vi "XML - Get General Settings.vi"(8 "error in (no error)":errorcluster, 11 "Target Ref in":T2 format="%.0x") -> (0 "error out":errorcluster, 2 "XML Header Data":T1, 3 "Target Ref out":T2 format="%.0x")   [LabVIEW 2019]
doc: "This VI gets all General Settings information required for the export to the XML File. It includes:\n- Custom-Device Type (Synchronous (UDP) - Asynchronous (TCP))\n- Controller Name\n- System Definition File Version\n- Creation Date."
uses:
  <vilib>/NI VeriStand/Custom Device API/Custom Device Item Ref.ctl
  Types/XML/XML - Header Data.ctl
  <vilib>/NI VeriStand/Custom Device API/Custom Device Pointer.ctl
  NationalInstruments.VeriStand.SystemStorage
  <vilib>/NI VeriStand/Custom Device API/Custom Device API.lvlib
  UDP-Custom-Device System Explorer.lvlib
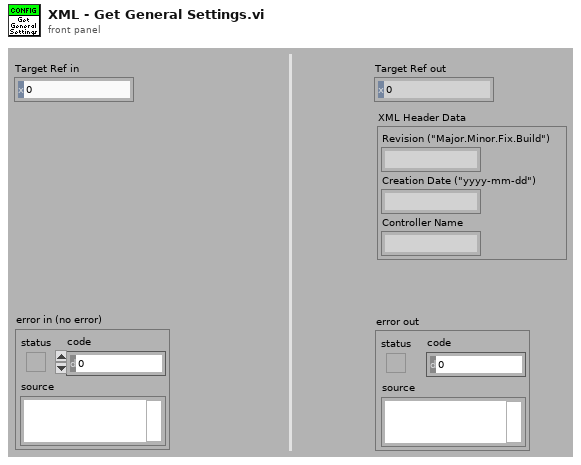
[diagram p1: front panel]
types:
  T1 = typedef "UDP-Custom-Device System Explorer.lvlib/XML - Header Data.ctl" = cluster{"Revision (\"Major.Minor.Fix.Build\")":string, "Creation Date (\"yyyy-mm-dd\")":string, "Controller Name":string}
  T2 = typedef "Custom Device API.lvlib/Custom Device Item Ref.ctl" = u64
  T3 = typedef "Custom Device API.lvlib/Custom Device Pointer.ctl" = refnum<k24>
  T4 = typedef "Custom Device API.lvlib/Custom Device Item Info.ctl" = cluster{"Name":string, "Is Channel":bool, "GUID":string, "Is Waveform":bool}
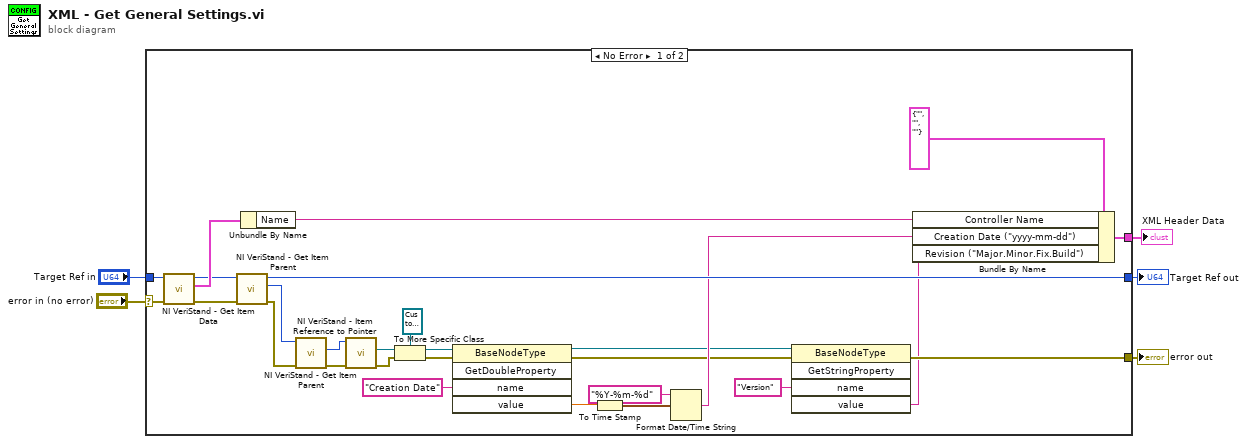
[diagram p0: block diagram]
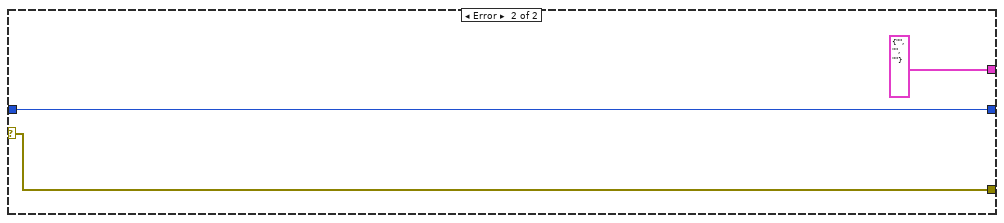
[diagram p2: hidden frame]
diagram:
  n1 = case shown="No Error" "error in (no error)" {
    selector: "error in (no error)" -> [w8 w35]
    tunnel: [w6 T1 {"Revision (\"Major.Minor.Fix.Build\")"="", "Creation Date (\"yyyy-mm-dd\")"="", "Controller Name"=""} ("XML Header Data")] -> w1
    tunnel: "Target Ref in" -> [w22 w36]
    tunnel: [w20 w36] -> w4
    tunnel: [w13 w35] -> w3
    frame No Error {
      n2 = call <vilib>:"NI VeriStand - Get Item Data.vi"("error in (no error)"=w8, "Item Ref in"=w22) -> ("error out"=w24:errorcluster, "Item Info"=w25:T4, "Item Ref out"=w23:T2)  [unwired: 6 in, 1 out]
      n3 = call <vilib>:"NI VeriStand - Get Item Parent.vi"("error in (no error)"=w24, "Item Ref in"=w23) -> ("error out"=w33:errorcluster, "Parent Ref"=w32:T2, "Item Ref out"=w20:T2)  [unwired: 6 in, 1 out]
      n4 = Unbundle By Name(w25) -> ("Name"=w21:string)
      n5 = call <vilib>:"NI VeriStand - Get Item Parent.vi"("error in (no error)"=w33, "Item Ref in"=w32) -> ("error out"=w31:errorcluster, "Parent Ref"=w30:T2)  [unwired: 6 in, 2 out]
      n6 = call <vilib>:"NI VeriStand - Item Reference to Pointer.vi"("error in (no error)"=w31, "Item Ref in"=w30) -> ("error out"=w14:errorcluster, "Node Pointer"=w29:T3)  [unwired: 6 in, 2 out]
      n7 = To More Specific Class(target class=T3 refnum ("reference"), reference=w29, error in=w14) -> (specific class reference=w26:T3, error out=w27:errorcluster)
      n8 = invoke class="BaseNodeType" method="GetDoubleProperty"(reference=w26, error in=w27, "name"="Creation Date") -> (reference out=w15:T3, error out=w9:errorcluster, "value"=w18:dbl)  [unwired: 2 in, 2 out]
      n9 = To Time Stamp(1:w18) -> (0:w17:timestamp)
      n10 = Format Date/Time String(time format string (%c)="%Y-%m-%d", seconds (now)=w17) -> (date/time string=w16:string)  [unwired: 1 in]
      n11 = invoke class="BaseNodeType" method="GetStringProperty"(reference=w15, error in=w9, "name"="Version") -> (error out=w13:errorcluster, "value"=w11:string)  [unwired: 2 in, 3 out]
      n12 = Bundle By Name(cluster=T1 {"Revision (\"Major.Minor.Fix.Build\")"="", "Creation Date (\"yyyy-mm-dd\")"="", "Controller Name"=""} ("XML Header Data"), "Controller Name"=w21, "Creation Date (\"yyyy-mm-dd\")"=w16, "Revision (\"Major.Minor.Fix.Build\")"=w11) -> (w6:T1)
    }
    frame Error {
    }
  }
  "error out" <- w3
  "Target Ref out" <- w4
  "XML Header Data" <- w1
